vi "Restart.HandleSequenceFinishedEvent.vi"(8 "error in (no error)":errorcluster, 10 "results path":path, 11 "State Variables":T1) -> (0 "error out":errorcluster)   [LabVIEW 2013, in "Simple Sequence Tools - Execution.lvlib"]
uses:
  Simple Sequence Tools - Execution.lvlib
  Types/Main.StateVariables.ctl
  Types/Execute.UserEventRefs.ctl
  <vilib>/NI Veristand/Execution/Workspace/SystemStateRegEventRef.ctl
  Types/Execution.SequenceState.ctl
  <vilib>/NI Veristand/Execution/DataLogging/DataLoggingSpecification Ref.ctl
  NationalInstruments.VeriStand.ClientAPI
  <vilib>/NI Veristand/Execution/DataLogging/IDataLogging Ref.ctl
  <vilib>/NI Veristand/Execution/Workspace/WorkspaceAPI.ctl
  NationalInstruments.VeriStand.RealTimeSequenceDefinitionApi
  <vilib>/NI Veristand/Execution/Workspace/SystemStateEventRef.ctl
  Shared/Types/INI.Settings
  <vilib>/NI Veristand/Execution/Workspace/NI VeriStand - Get Single Channel Value.vi
  <vilib>/NI Veristand/Execution/Workspace/NI_VS Workspace ExecutionAPI.lvlib
  <vilib>/NI Veristand/Execution/DataLogging/NI_VS Data Logging API.lvlib
  Shared/Simple Sequence Tools - Shared.lvlib
panel:
  out "State Variables out":T1
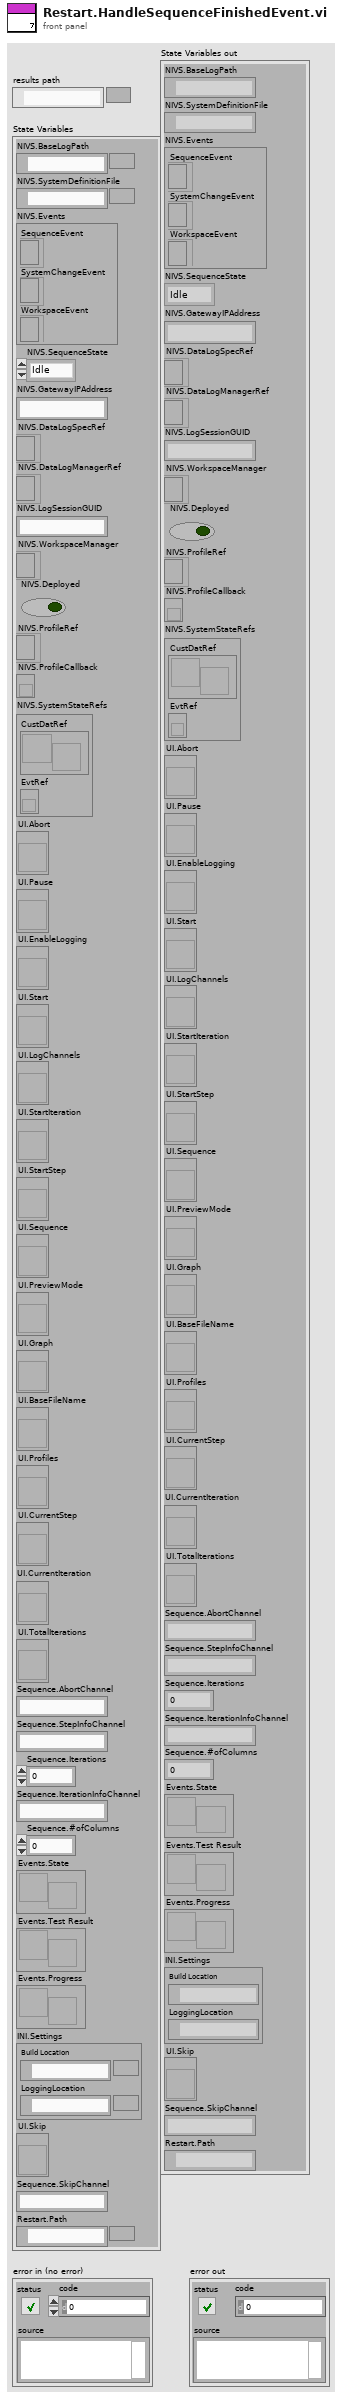
[diagram p1: front panel]
types:
  T1 = typedef "Simple Sequence Tools - Execution.lvlib/Main.StateVariables.ctl" = cluster{"NIVS.BaseLogPath":path, "NIVS.SystemDefinitionFile":path, "NIVS.Events":T2, "NIVS.SequenceState":T4, "NIVS.GatewayIPAddress":string, "NIVS.DataLogSpecRef":T5, "NIVS.DataLogManagerRef":T6, "NIVS.LogSessionGUID":string, "NIVS.WorkspaceManager":T7, "NIVS.Deployed":bool, "NIVS.ProfileRef":refnum<k24>, "NIVS.ProfileCallback":refnum<k27>, "NIVS.SystemStateRefs":T8, "UI.Abort":refnum<vi>, "UI.Pause":refnum<vi>, "UI.EnableLogging":refnum<vi>, "UI.Start":refnum<vi>, "UI.LogChannels":refnum<vi>, "UI.StartIteration":refnum<vi>, "UI.StartStep":refnum<vi>, "UI.Sequence":refnum<vi>, "UI.PreviewMode":refnum<vi>, "UI.Graph":refnum<vi>, "UI.BaseFileName":refnum<vi>, "UI.Profiles":refnum<vi>, "UI.CurrentStep":refnum<vi>, "UI.CurrentIteration":refnum<vi>, "UI.TotalIterations":refnum<vi>, "Sequence.AbortChannel":string, "Sequence.StepInfoChannel":string, "Sequence.Iterations":u32, "Sequence.IterationInfoChannel":string, "Sequence.#ofColumns":i32, "Events.State":refnum<user-event>, "Events.Test Result":refnum<user-event>, "Events.Progress":refnum<user-event>, "INI.Settings":T9, "UI.Skip":refnum<vi>, "Sequence.SkipChannel":string, "Restart.Path":path}
  T2 = typedef "Simple Sequence Tools - Execution.lvlib/Execute.UserEventRefs.ctl" = cluster{"SequenceEvent":refnum<event-registration>, "SystemChangeEvent":T3, "WorkspaceEvent":refnum<event-registration>}
  T3 = typedef "NI_VS Workspace ExecutionAPI.lvlib/SystemStateRegEventRef.ctl" = refnum<event-registration>
  T4 = typedef "Simple Sequence Tools - Execution.lvlib/Execution.SequenceState.ctl" = enum16{"Idle", "Initializing", "Running", "Paused", "Finalizing", "Complete"}
  T5 = typedef "NI_VS Data Logging API.lvlib/DataLoggingSpecification Ref.ctl" = refnum<k24>
  T6 = typedef "NI_VS Data Logging API.lvlib/IDataLogging Ref.ctl" = refnum<k24>
  T7 = typedef "NI_VS Workspace ExecutionAPI.lvlib/WorkspaceAPI.ctl" = refnum<k24>
  T8 = typedef "NI_VS Workspace ExecutionAPI.lvlib/SystemStateEventRef.ctl" = cluster{"CustDatRef":refnum<user-event>, "EvtRef":refnum<k27>}
  T9 = typedef "Simple Sequence Tools - Shared.lvlib/INI.Settings" = cluster{"Build Location":path, "LoggingLocation":path}
  T10 = typedef "Simple Sequence Tools - Execution.lvlib/Results.Value.ctl" = enum8{"Passed", "Failed", "Aborted"}
  T11 = typedef "Simple Sequence Tools - Execution.lvlib/Restart.Settings" = cluster{"LogFile":path, "Log Settings":T12[], "StimulusProfile":path, "StopIteration":i32, "StopStep":i32, "Log Channels":T16, "Base File Name":string, "Enable Logging":bool, "Profiles":string}
  T12 = typedef "NI_VS Data Logging API.lvlib/TDMS Channel Group.ctl" = cluster{"Group Name":string, "Group Description":string, "Group Properties":T13[], "Channels":T14[], "Time Channel Options":T15, "Time Channel Name":string}
  T13 = typedef "NI_VS Data Logging API.lvlib/TDMS Property.ctl" = cluster{"Name":string, "Value":variant}
  T14 = typedef "NI_VS Data Logging API.lvlib/TDMS Channel.ctl" = cluster{"Channel Name":string, "Channel Path":string, "Channel Description":string, "Channel Properties":T13[]}
  T15 = typedef "NI_VS Data Logging API.lvlib/Time Channel Options.ctl" = enum16{"No Time Channel", "Absolute Time", "System Time", "System Time - Microseconds", "Absolute Time as Double"}
  T16 = typedef "Simple Sequence Tools - Execution.lvlib/Log.SelectedChannels.ctl" = enum16{"Channels (No System Channel)", "Aliases", "All"}
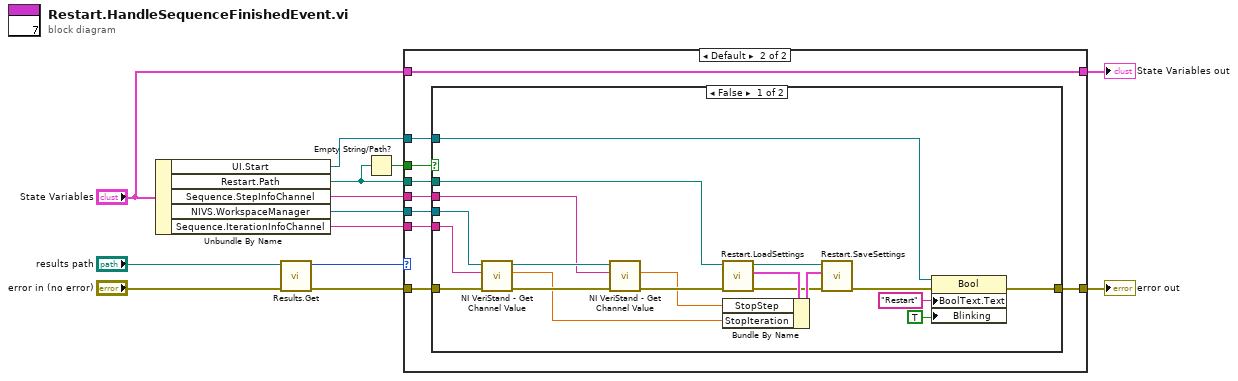
[diagram p0: block diagram]
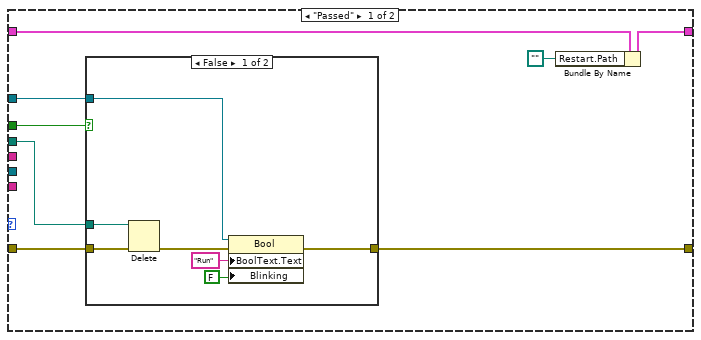
[diagram p2: hidden frame]
diagram:
  n1 = Unbundle By Name("State Variables") -> ("UI.Start"=w1:refnum<vi>, "Restart.Path"=w8:path, "Sequence.StepInfoChannel"=w7:string, "NIVS.WorkspaceManager"=w5:T7, "Sequence.IterationInfoChannel"=w6:string)
  n2 = call "Results.Get.vi"("error in (no error)"="error in (no error)", "path"="results path") -> ("error out"=w10:errorcluster, "Result"=w9:T10)  [unwired: 8 in]
  n3 = Empty String/Path?(string/path=w8) -> (empty?=w4:bool)
  n4 = case shown="Default" w9 {
    tunnel: w4 -> [w21 w38]
    tunnel: w5 -> [_ w37]
    tunnel: w6 -> [_ w36]
    tunnel: w7 -> [_ w35]
    tunnel: w8 -> [w20 w34]
    tunnel: w10 -> [w19 w33]
    tunnel: [w18 w32] -> w11
    tunnel: "State Variables" -> [w17 w31]
    tunnel: [w15 w31] -> w2
    tunnel: w1 -> [w14 w30]
    frame "Passed" {
      n5 = case shown="False" w21 {
        tunnel: w19 -> [w28 w29]
        tunnel: [w22 w29] -> w18
        tunnel: w20 -> [w27 _]
        tunnel: w14 -> [w24 _]
        frame False {
          n6 = Delete(path (use dialog)=w27, error in=w28) -> (error out=w23:errorcluster)  [unwired: 3 in, 2 out]
          n7 = property class="Bool"(reference=w24, error in=w23, "BoolText.Text"="Run" ("Boolean Text.Text"), "Blinking"=FALSE) -> (error out=w22:errorcluster)  [unwired: 1 out]
        }
        frame True {
        }
      }
      n8 = Bundle By Name(cluster=w17, "Restart.Path"=path "") -> (w15:T1)
    }
    frame Default {
      n9 = case shown="False" w38 {
        tunnel: w34 -> [w54 _]
        tunnel: w37 -> [w53 _]
        tunnel: w36 -> [w51 _]
        tunnel: w35 -> [w50 _]
        tunnel: [w42 w58] -> w32
        tunnel: w33 -> [w44 w58]
        tunnel: w30 -> [w41 _]
        frame False {
          n10 = call-poly <vilib>:"NI VeriStand - Get Channel Value.vi"("error in (no error)"=w44, "Channel"=w51, "WorkspaceManager in"=w53) -> ("error out"=w49:errorcluster, "Value"=w45:dbl, "WorkspaceManager out"=w52:T7)  [unwired: 6 in]
          n11 = call-poly <vilib>:"NI VeriStand - Get Channel Value.vi"("error in (no error)"=w49, "Channel"=w50, "WorkspaceManager in"=w52) -> ("error out"=w48:errorcluster, "Value"=w46:dbl)  [unwired: 6 in, 1 out]
          n12 = call "Restart.LoadSettings.vi"("error in"=w48, "datalog path (use dialog)"=w54) -> ("error out"=w47:errorcluster, "Restart Settings"=w56:T11, "path"=w57:path)  [unwired: 7 in]
          n13 = Bundle By Name(cluster=w56, "StopStep"=w46, "StopIteration"=w45) -> (w55:T11)
          n14 = call "Restart.SaveSettings.vi"("error in"=w47, "Restart Settings"=w55, "datalog path (use dialog)"=w57) -> ("error out"=w43:errorcluster)  [unwired: 7 in, 1 out]
          n15 = property class="Bool"(reference=w41, error in=w43, "BoolText.Text"="Restart" ("Boolean Text.Text"), "Blinking"=TRUE) -> (error out=w42:errorcluster)  [unwired: 1 out]
        }
        frame True {
        }
      }
    }
  }
  "error out" <- w11
  "State Variables out" <- w2
